vi "ToscaTTL-Pulse Output.vi"(0 "task in":refnum<k21>, 5 "StopWhen":string, 7 "StopValue":dbl, 9 "Pulse":T1, 11 "error in (no error)":errorcluster, 13 "TTL Queue":refnum<queue>) -> (4 "task out":refnum<k21>, 8 "trigger":bool, 15 "error out":errorcluster)   [LabVIEW 2020]
uses:
  Control Classes/Base Class/TTLController.lvclass
  <vilib>/DAQmx/write.llb/DAQmx Write (Digital Bool 1Line 1Point).vi
  <vilib>/DAQmx/miscellaneous.llb/DAQmx Fill In Error Info.vi
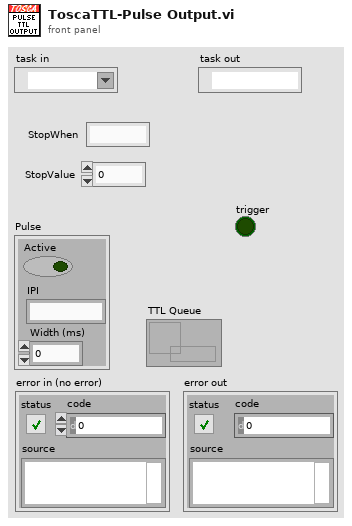
[diagram p1: front panel]
types:
  T1 = cluster{"Active":bool, "IPI":string, "Width (ms)":dbl}
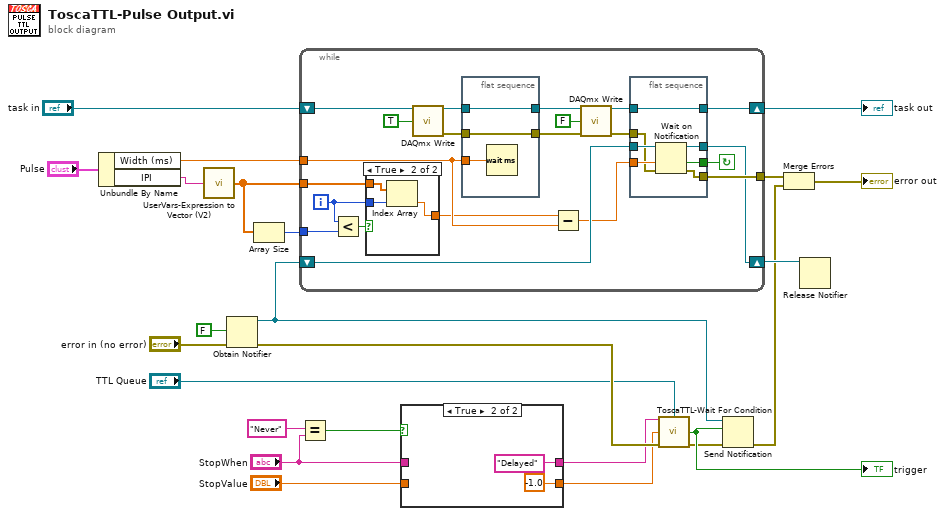
[diagram p0: block diagram]
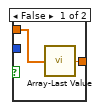
[diagram p3: hidden frame]
diagram:
  n1 = Unbundle By Name("Pulse") -> ("Width (ms)"=w10:dbl, "IPI"=w1:string)
  n2 = call "UserVars-Expression to Vector (V2).vi"("Expr"=w1) -> ("Values"=w3:dbl[])  [unwired: 13 in, 1 out]
  n3 = Obtain Notifier(notification data type=FALSE, error in (no error)="error in (no error)") -> (notifier out=w18:refnum<notifier>, error out=w15:errorcluster)  [unwired: 2 in, 1 out]
  n4 = Array Size(array=w3) -> (size(s)=w2:i32)
  n5 = while {
    tunnel: w10 -> [w31]
    tunnel: [w35] -> w19
    shift-right: [w34] -> w22
    shift-left: "task in" -> [w33]
    shift-right: [w32] -> w24
    shift-left: w18 -> [w37]
    tunnel: w3 -> [w26]
    tunnel: w2 -> [w29]
    i -> [w28]
    stop <- w36 continue-if-true
    n6 = Less?(x=w28, y=w29) -> (x < y?=w27:bool)
    n7 = case shown="True" w27 {
      tunnel: w28 -> [_ w49]
      tunnel: w26 -> [w46 w50]
      tunnel: [w47 w48] -> w25
      frame False {
        n8 = call "Array-Last Value.vi"("array"=w46) -> ("element"=w47:dbl)
      }
      frame True {
        n9 = Index Array(array=w50, index=w49) -> (element=w48:dbl)
      }
    }
    n10 = call-poly <vilib>:"DAQmx Write.vi"("task/channels in"=w33, "data"=TRUE) -> ("task out"=w39:refnum<k21>, "error out"=w44:errorcluster)  [unwired: 11 in, 1 out]
    n11 = flat-sequence {
      tunnel: w44 -> [w60]
      tunnel: [w60] -> w41
      tunnel: [w59] -> w40
      tunnel: w39 -> [w59]
      tunnel: w31 -> [w58]
      frame #0 {
        n12 = Wait (ms)(milliseconds to wait=w58) -> ()  [unwired: 1 out]
      }
    }
    n13 = Subtract(x=w25, y=w31) -> (x-y=w30:dbl)
    n14 = call-poly <vilib>:"DAQmx Write.vi"("task/channels in"=w40, "data"=FALSE, "error in"=w41) -> ("task out"=w38:refnum<k21>, "error out"=w42:errorcluster)  [unwired: 10 in, 1 out]
    n15 = flat-sequence {
      tunnel: w42 -> [w53]
      tunnel: w38 -> [w57]
      tunnel: [w57] -> w34
      tunnel: w30 -> [w56]
      tunnel: w37 -> [w55]
      tunnel: [w54] -> w36
      tunnel: [w52] -> w35
      tunnel: [w51] -> w32
      frame #0 {
        n16 = Wait on Notification(notifier=w55, timeout in ms (-1)=w56, error in (no error)=w53) -> (notifier out=w51:refnum<notifier>, timed out?=w54:bool, error out=w52:errorcluster)  [unwired: 1 in, 1 out]
      }
    }
  }
  "task out" <- w22
  n17 = Equal?(x="Never" ("y"), y="StopWhen") -> (x = y?=w14:bool)
  n18 = case shown="True" w14 {
    tunnel: [w62 "Delayed" ("When")] -> w7
    tunnel: "StopWhen" -> [w62 _]
    tunnel: "StopValue" -> [w61 _]
    tunnel: [w61 -1.0 ("Value")] -> w4
    frame False {
    }
    frame True {
    }
  }
  n19 = call "ToscaTTL-Wait For Condition.vi"("When"=w7, "Control Queue"="TTL Queue", "Value"=w4, "error in (no error)"=w15) -> ("trigger"=w17:bool, "error out"=w16:errorcluster)  [unwired: 10 in]
  "trigger" <- w17
  n20 = Send Notification(notification=w17, notifier=w18, error in (no error)=w16) -> (error out=w20:errorcluster)  [unwired: 1 out]
  n21 = Merge Errors(w19, w20) -> (→"error out":errorcluster)
  n22 = Release Notifier(notifier=w24) -> ()  [unwired: 2 in, 3 out]
